vi "test-trapezoid-profile-timing-to-current.vi"() -> (3 "Test Passed":bool)   [LabVIEW 2019]
uses:
  <vilib>/Rock Robotics/WPI/ThirdParty/JAS_Junk/TrajLib/TRAPEZOID_PROFILE_STATE.ctl
  <vilib>/Rock Robotics/WPI/ThirdParty/JAS_Junk/TrajLib/TRAPEZOID_PROFILE.ctl
  <vilib>/Rock Robotics/WPI/ThirdParty/JAS_Junk/TrajLib/TRAPEZOID_PROFILE_CONSTRAINT.ctl
  <vilib>/Rock Robotics/WPI/ThirdParty/JAS_Junk/TrajLib/TrapProfile_ShouldFlipAcceleration.vi
  <vilib>/Rock Robotics/WPI/ThirdParty/JAS_Junk/TrajLib/TrapProfile_Direct.vi
  <vilib>/Rock Robotics/SystemInterfaces/NetworkCommunication/NetComm_UsageReport_report.vi
  <vilib>/Rock Robotics/WPI/ThirdParty/JAS_Junk/TrajLib/Util_LibraryGlobals.vi
  <vilib>/Rock Robotics/WPI/ThirdParty/JAS_Junk/TrajLib/Trajectory_Library.lvlib
panel:
  out "ApproxEquals 2":bool
  out "ApproxEquals":bool
  out "Equal 2":bool
  out "TimeLeftGoal":dbl
  out "TimeLeftPos":dbl
  out "Equal":bool
  out "TotalTime":dbl
  out "TRAPEZOID_PROFILE":T1 {"Goal"."Velocity" format="%16_6e"; "Goal"."Position" format="%16_6e"; "Initial"."Velocity" format="%16_6e"; "Initial"."Position" format="%16_6e"; "Constraints"."MaxAcceleration" format="%16_6e"; "Constraints"."MaxVelocity" format="%16_6e"; "EndDecel" format="%16_6e"; "EndFullSpeed" format="%16_6e"; "EndAccel" format="%16_6e"}
  out "State":T3 {"Velocity" format="%16_6e"; "Position" format="%16_6e"}
  out "Waveform Chart":T4(graph)
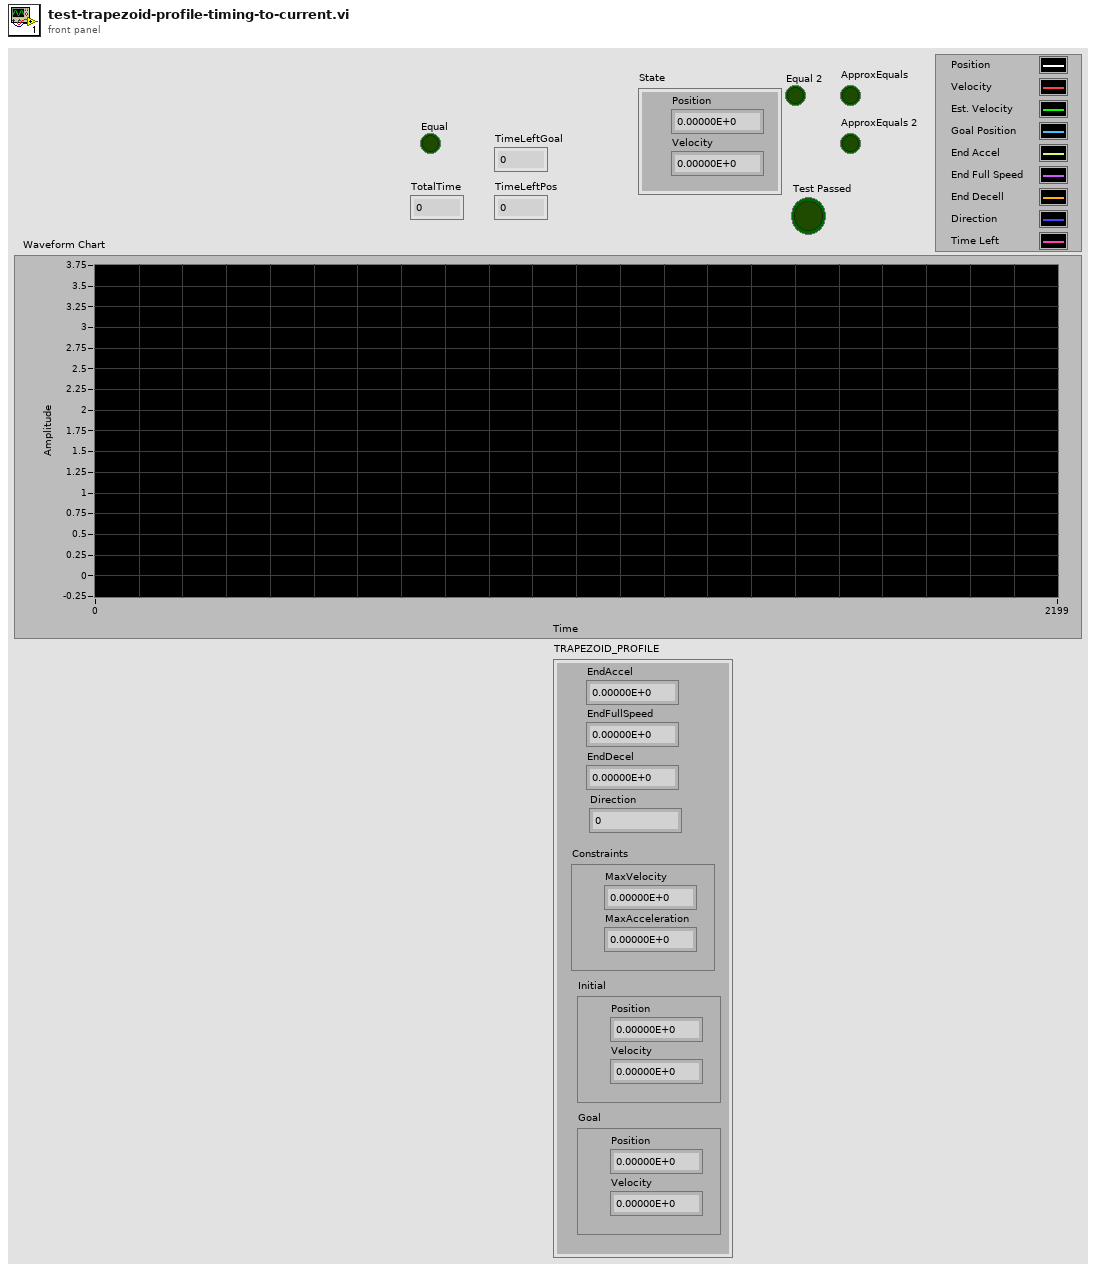
[diagram p1: front panel]
types:
  T1 = typedef "Trajectory_Library.lvlib/TRAPEZOID_PROFILE.ctl" = cluster{"EndAccel":dbl, "EndFullSpeed":dbl, "EndDecel":dbl, "Direction":i32, "Constraints":T2, "Initial":T3, "Goal":T3}
  T2 = typedef "Trajectory_Library.lvlib/TRAPEZOID_PROFILE_CONSTRAINT.ctl" = cluster{"MaxVelocity":dbl, "MaxAcceleration":dbl}
  T3 = typedef "Trajectory_Library.lvlib/TRAPEZOID_PROFILE_STATE.ctl" = cluster{"Position":dbl, "Velocity":dbl}
  T4 = cluster{"Position":dbl, "Velocity":dbl, dbl, "Position":dbl, "EndAccel":dbl, "EndFullSpeed":dbl, "EndDecel":dbl, "Direction":i32, "Position":dbl}
  T5 = cluster{"Position":dbl, "Velocity":dbl, dbl, "Position":dbl, "EndAccel":dbl, "EndFullSpeed":dbl, "EndDecel":dbl, "Direction":i32, "TimeLeft":dbl}
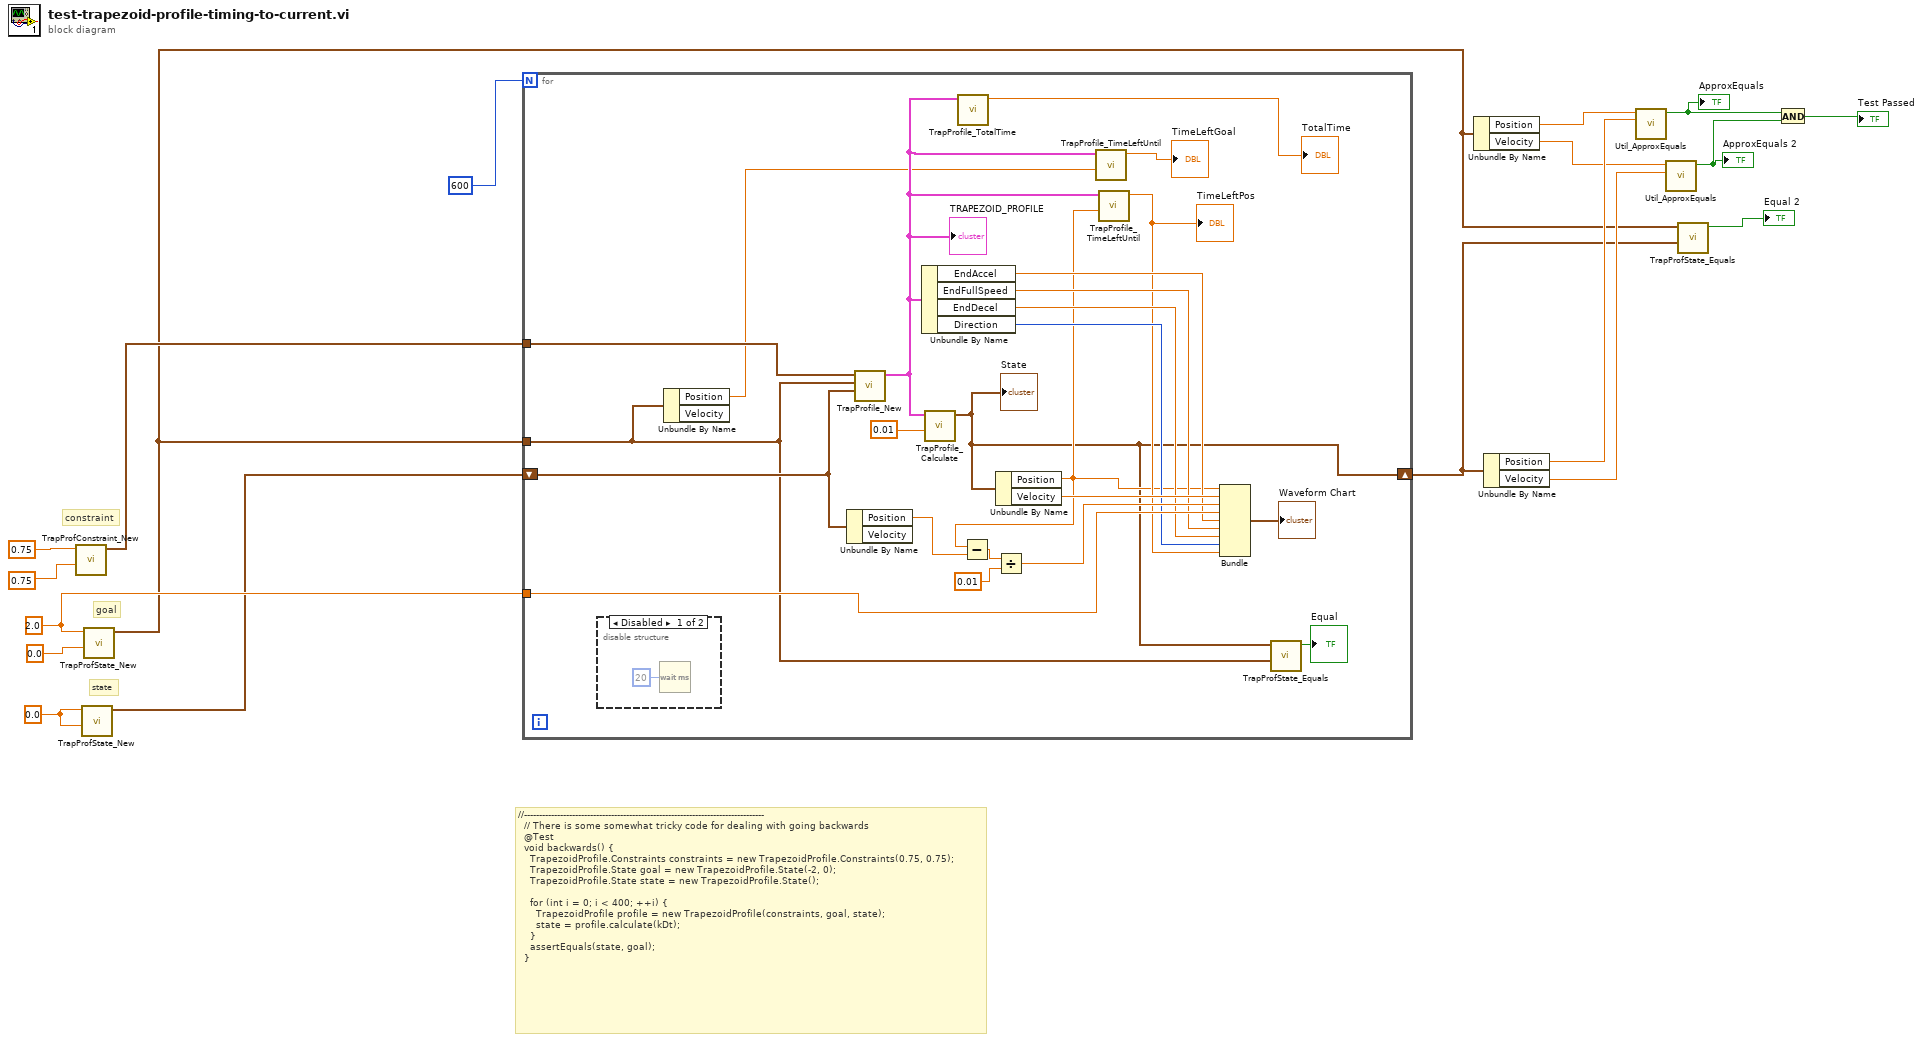
[diagram p0: block diagram]
diagram:
  w12 = 0.0 ("Position")
  w13 = 2.0 ("Position")
  # "state"
  # "//--------------------------------------------------------------------------------\n  // There is some somewhat tricky code for dealing with going backwards\n  @Test\n  void backwards() {\n    TrapezoidProfile.Constraints constraints = new TrapezoidProfile.Constraints(0.75, 0.75);\n    TrapezoidProfile.State goal = new TrapezoidProfile.State(-2, 0);\n    TrapezoidProfile.State state = new TrapezoidProfile.State();\n\n    for (int i = 0; i < 400; ++i) {\n      TrapezoidProfile profile = new TrapezoidProfile(constraints, goal, state);\n      state = profile.calculate(kDt);\n    }\n    assertEquals(state, goal);\n  }"
  # "goal"
  # "constraint"
  n1 = call <vilib>:"TrapProfConstraint_New.vi"("Max Accel"=0.75, "Max Speed (M/S)"=0.75) -> ("TRAPEZOID_PROFILE_CONSTRAINT"=w14:T2)  [unwired: 9 in]
  n2 = call <vilib>:"TrapProfState_New.vi"("Velocity"=w12, "Position"=w12) -> ("TRAPEZOID_PROFILE_STATE"=w11:T3)  [unwired: 9 in]
  n3 = call <vilib>:"TrapProfState_New.vi"("Velocity"=0.0, "Position"=w13) -> ("TRAPEZOID_PROFILE_STATE"=w1:T3)  [unwired: 9 in]
  n4 = for {
    N: 600 -> [_]
    shift-right: [w24] -> w2
    shift-left: w11 -> [w38]
    tunnel: w1 -> [w20]
    tunnel: w13 -> [w34]
    tunnel: w14 -> [w28]
    n5 = disable-structure shown="Disabled" {
      frame Disabled {
        n6 = Wait (ms)(milliseconds to wait=u32 20) -> ()  [unwired: 1 out]
      }
      frame Enabled {
      }
    }
    n7 = Unbundle By Name(w20) -> ("Position"=w19:dbl)  [unwired: 1 out]
    n8 = Unbundle By Name(w38) -> ("Position"=w29:dbl)  [unwired: 1 out]
    n9 = call <vilib>:"TrapProfile_New.vi"("Initial"=w38, "Goal"=w20, "Constraints"=w28) -> ("TRAPEZOID_PROFILE"=w22:T1)  [unwired: 8 in]
    "TRAPEZOID_PROFILE" <- w22
    n10 = Unbundle By Name(w22) -> ("EndAccel"=w33:dbl, "EndFullSpeed"=w32:dbl, "EndDecel"=w31:dbl, "Direction"=w30:i32)
    n11 = call <vilib>:"TrapProfile_Calculate.vi"("Time"=0.01, "TRAPEZOID_PROFILE"=w22) -> ("State"=w24:T3)  [unwired: 9 in]
    "State" <- w24
    n12 = call <vilib>:"TrapProfile_TotalTime.vi"("TRAPEZOID_PROFILE"=w22) -> ("TotalTime"=→"TotalTime":dbl)  [unwired: 10 in]
    n13 = Unbundle By Name(w24) -> ("Position"=w26:dbl, "Velocity"=w40:dbl)
    n14 = Subtract(x=w26, y=w29) -> (x-y=w37:dbl)
    n15 = Divide(x=w37, y=0.01) -> (x/y=w35:dbl)
    n16 = call <vilib>:"TrapProfile_TimeLeftUntil.vi"("TargetDistance"=w19, "TRAPEZOID_PROFILE"=w22) -> ("TimeLeft"=→"TimeLeftGoal":dbl)  [unwired: 9 in]
    n17 = call <vilib>:"TrapProfile_TimeLeftUntil.vi"("TargetDistance"=w26, "TRAPEZOID_PROFILE"=w22) -> ("TimeLeft"=w27:dbl)  [unwired: 9 in]
    "TimeLeftPos" <- w27
    n18 = Bundle("Position"=w26, "Velocity"=w40, w35, "Position"=w34, "EndAccel"=w33, "EndFullSpeed"=w32, "EndDecel"=w31, "Direction"=w30, "TimeLeft"=w27) -> (→"Waveform Chart":T5)  [unwired: 1 in]
    n19 = call <vilib>:"TrapProfState_Equals.vi"("TRAPEZOID_PROFILE_STATE 2"=w20, "TRAPEZOID_PROFILE_STATE"=w24) -> ("Equal"=→"Equal":bool)  [unwired: 9 in]
  }
  n20 = Unbundle By Name(w1) -> ("Position"=w10:dbl, "Velocity"=w8:dbl)
  n21 = Unbundle By Name(w2) -> ("Position"=w9:dbl, "Velocity"=w6:dbl)
  n22 = call <vilib>:"Util_ApproxEquals.vi"("Value 2"=w9, "Value 1"=w10) -> ("ApproxEquals"=w4:bool)  [unwired: 9 in]
  "ApproxEquals" <- w4
  n23 = call <vilib>:"Util_ApproxEquals.vi"("Value 2"=w6, "Value 1"=w8) -> ("ApproxEquals"=w3:bool)  [unwired: 9 in]
  "ApproxEquals 2" <- w3
  n24 = call <vilib>:"TrapProfState_Equals.vi"("TRAPEZOID_PROFILE_STATE 2"=w2, "TRAPEZOID_PROFILE_STATE"=w1) -> ("Equal"=→"Equal 2":bool)  [unwired: 9 in]
  n25 = And(x=w4, y=w3) -> (x .and. y?=→"Test Passed":bool)
